vi "test Add-Get-Remove Port and Port Number.vi"(8 "error in":errorcluster, 11 "TestCase in":refnum<class "Scripting.lvclass">) -> (0 "error out":errorcluster, 3 "TestCase out":refnum<class "Scripting.lvclass">)   [LabVIEW 2020, in "Scripting.lvclass"]
uses:
  Scripting.lvclass
  C:/dev/git/niveristand-custom-device-testing-tools/VeriStandScriptingTestCase/VeriStandScriptingTestCase.lvclass
  <vilib>/NI VeriStand/Custom Device API/Custom Device Item Ref.ctl
  niveristand-custom-device-testing-tools/VeriStandScriptingTestCase/VeriStandScriptingTestCase.lvclass/VeriStandScriptingTestCase.ctl
  niveristand-custom-device-testing-tools/VeriStandScriptingTestCase/Read Target.vi
  NationalInstruments.VeriStand.SystemDefinitionAPI
  <vilib>/addons/_JKI Toolkits/VI Tester/TestCase.llb/TestCase.lvclass
  Scripting/AIM MIL-STD-1553 Scripting.lvlib
  <vilib>/NI VeriStand/Custom Device API/Custom Device API.lvlib
  C:/Program Files (x86)/National Instruments/LabVIEW 2020/vi.lib/addons/_JKI Toolkits/VI Tester/TestCase.llb/TestCase.lvclass
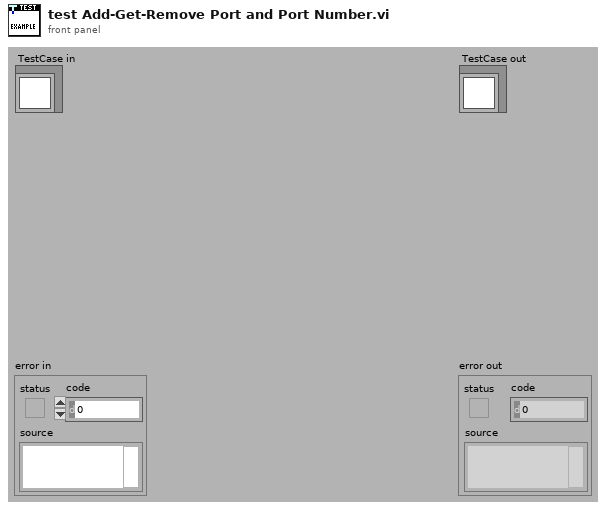
[diagram p1: front panel]
types:
  T1 = typedef "Custom Device API.lvlib/Custom Device Item Ref.ctl" = u64
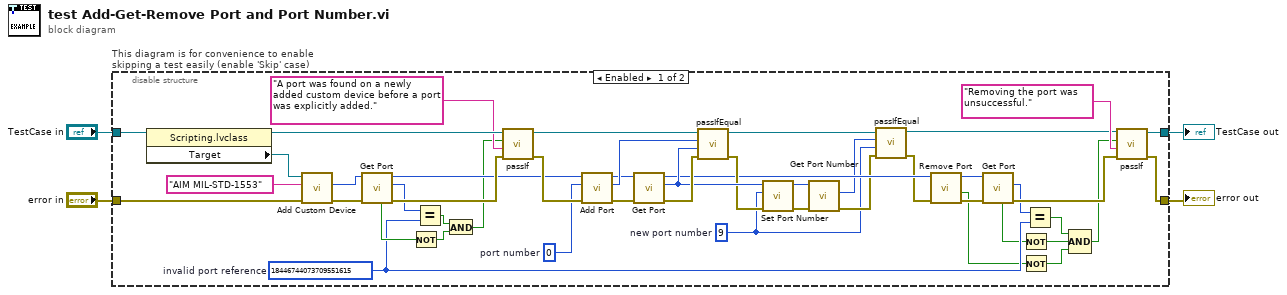
[diagram p0: block diagram]
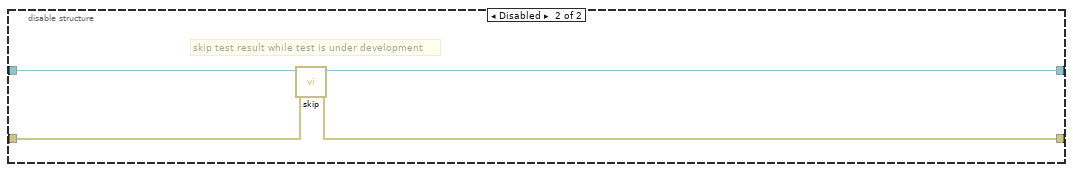
[diagram p2: hidden frame]
diagram:
  n1 = disable-structure "This diagram is for convenience to enable skipping a test easily (enable 'Skip' case)" shown="Enabled" {
    disable-tunnel: "TestCase in" -> [w49 w55]
    disable-tunnel: [w36 w53] -> w1
    disable-tunnel: [w37 w54] -> w3
    disable-tunnel: "error in" -> [w51 w52]
    frame Enabled {
      w13 = u16 9  # new port number
      w11 = T1 18446744073709551615  # invalid port reference
      w41 = 0  # port number
      n2 = property class="Scripting.lvclass"(reference=w49) -> (reference out=w47:refnum<class "Scripting.lvclass">, "Target"=w48:refnum<k24>)  [unwired: 1 in, 1 out]
      n3 = call "Add Custom Device.vi"("error in"=w51, "custom device name"="AIM MIL-STD-1553" ("name"), "target"=w48) -> ("error out"=w35:errorcluster, "custom device ref out"=w32:T1)  [unwired: 6 in, 1 out]
      n4 = call "Get Port.vi"("error in"=w35, "custom device ref"=w32) -> ("error out"=w34:errorcluster, "port"=w31:T1, "custom device ref out"=w33:T1, "found"=w20:bool)  [unwired: 6 in]
      n5 = Not(x=w20) -> (.not. x?=w19:bool)
      n6 = Equal?(x=w31, y=w11) -> (x = y?=w21:bool)
      n7 = And(x=w21, y=w19) -> (x .and. y?=w22:bool)
      n8 = call-dynamic "passIf.vi"("error in (no error)"=w34, "message (\"\")"="A port was found on a newly added custom device before a port was explicitly added." ("message (\"\")"), "pass"=w22, "TestCase in"=w47) -> ("error out"=w46:errorcluster, "TestCase out"=w45:refnum<class "Scripting.lvclass">)  [unwired: 6 in]
      n9 = call "Add Port.vi"("error in"=w46, "port number"=w41, "custom device ref"=w33) -> ("error out"=w43:errorcluster, "port"=w44:T1, "custom device ref out"=w42:T1)  [unwired: 6 in]
      n10 = call "Get Port.vi"("error in"=w43, "custom device ref"=w42) -> ("error out"=w40:errorcluster, "port"=w28:T1, "custom device ref out"=w24:T1)  [unwired: 6 in, 1 out]
      n11 = call-dynamic "passIfEqual.vi"("error in (no error)"=w40, "y"=w28, "x"=w44, "TestCase in"=w45) -> ("error out"=w27:errorcluster, "TestCase out"=w18:refnum<class "Scripting.lvclass">)  [unwired: 6 in]
      n12 = call "Set Port Number.vi"("error in"=w27, "port number"=w13, "port"=w28) -> ("error out"=w26:errorcluster, "port out"=w25:T1)  [unwired: 7 in]
      n13 = call "Get Port Number.vi"("error in"=w26, "port"=w25) -> ("error out"=w16:errorcluster, "port number"=w14:u16)  [unwired: 6 in, 2 out]
      n14 = call-dynamic "passIfEqual.vi"("error in (no error)"=w16, "y"=w13, "x"=w14, "TestCase in"=w18) -> ("error out"=w15:errorcluster, "TestCase out"=w17:refnum<class "Scripting.lvclass">)  [unwired: 6 in]
      n15 = call "Remove Port.vi"("error in"=w15, "custom device ref"=w24) -> ("error out"=w39:errorcluster, "no port found"=w6:bool, "custom device ref out"=w23:T1)  [unwired: 7 in]
      n16 = call "Get Port.vi"("error in"=w39, "custom device ref"=w23) -> ("error out"=w38:errorcluster, "port"=w9:T1, "found"=w10:bool)  [unwired: 6 in, 1 out]
      n17 = Not(x=w10) -> (.not. x?=w7:bool)
      n18 = Not(x=w6) -> (.not. x?=w5:bool)
      n19 = Equal?(x=w9, y=w11) -> (x = y?=w12:bool)
      n20 = Compound Arithmetic op=AND(w12, w7, w5) -> (w8:bool)
      n21 = call-dynamic "passIf.vi"("error in (no error)"=w38, "message (\"\")"="Removing the port was unsuccessful." ("message (\"\")"), "pass"=w8, "TestCase in"=w17) -> ("error out"=w37:errorcluster, "TestCase out"=w36:refnum<class "Scripting.lvclass">)  [unwired: 6 in]
    }
    frame Disabled {
      # "skip test result while test is under development"
      n22 = call <vilib>:"skip.vi"("error in (no error)"=w52, "TestCase in"=w55) -> ("error out"=w54:errorcluster, "TestCase out"=w53:refnum<class "Scripting.lvclass">)  [unwired: 8 in]
    }
  }
  "error out" <- w3
  "TestCase out" <- w1
